vi "Controlled voltage ramp checking current.vi"(8 "V Ch 1":refnum<vi>, 9 "V Ch 0":refnum<vi>, 10 "Barcodes in":string[](array[string]), 11 "VISA Refnum in":refnum<visa-resource-name>) -> (0 "Ch 4 High":dbl[](array[numeric]), 1 "Ch 3 High":dbl[](array[numeric]), 2 "Ch 2 High":dbl[](array[numeric]), 3 "Ch 1 High":dbl[](array[numeric]), 4 "error out":errorcluster, 5 "BoardHandle out 3":T1, 6 "Current High":bool, 7 "Power Trip":bool)   [LabVIEW 2020]
uses:
  <instrlib>/CAEN PSM/CAEN PSM.lvlib
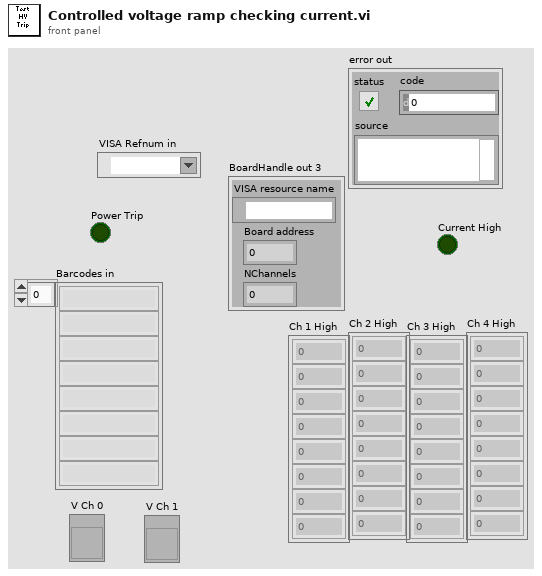
[diagram p1: front panel]
types:
  T1 = cluster{"VISA resource name":refnum<visa-resource-name>, "Board address":u8, "NChannels":u8}
  T2 = typedef "CAEN PSM.lvlib/BoardHandle.ctl" = cluster{"VISA resource name":refnum<visa-resource-name>, "Board address":i8, "NChannels":u8}
  T3 = cluster{"ON":bool, "RUP":bool, "RDW":bool, "OVC":bool, "OVV":bool, "UNV":bool, "MAXV":bool, "TRIP":bool, "OVP":bool, "OVT":bool, "DIS":bool, "KILL":bool, "ILK":bool, "NOCAL":bool}[]
  T4 = cluster{"ON":bool, "RUP":bool, "RDW":bool, "OVC":bool, "OVV":bool, "UNV":bool, "MAXV":bool, "TRIP":bool, "OVP":bool, "OVT":bool, "DIS":bool, "KILL":bool, "ILK":bool, "NOCAL":bool}
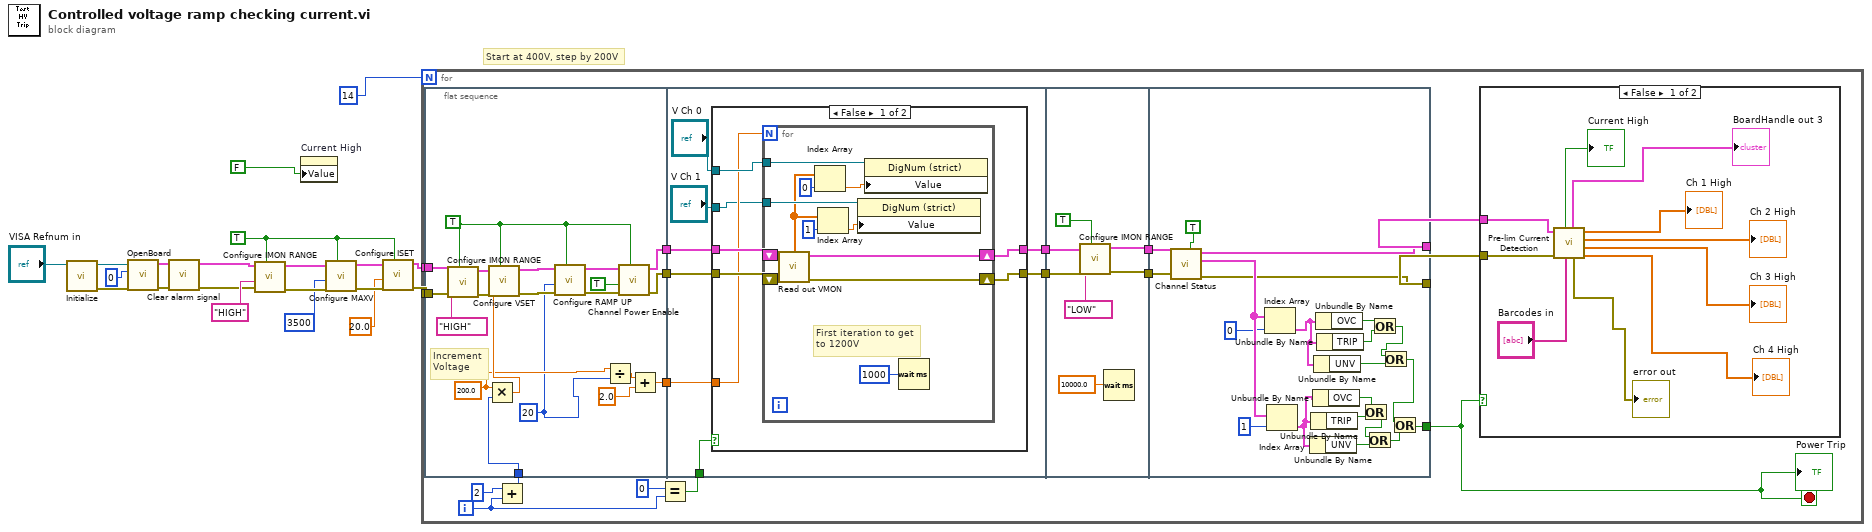
[diagram p0: block diagram]
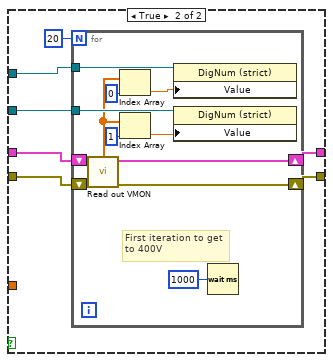
[diagram p3: hidden frame]
diagram:
  w6 = TRUE ("All Channels (F)")
  # "Start at 400V, step by 200V"
  n1 = call <instrlib>:"Initialize.vi"("VISA resource name"="VISA Refnum in") -> ("error out"=w17:errorcluster, "VISA resource name out"=w18:refnum<visa-resource-name>)  [unwired: 9 in]
  n2 = call <instrlib>:"OpenBoard.vi"("error in (no error)"=w17, "Board Address"=u8 0, "VISA resource name"=w18) -> ("error out"=w16:errorcluster, "BoardHandle"=w19:T2)  [unwired: 7 in]
  n3 = call <instrlib>:"Clear alarm signal.vi"("error in (no error)"=w16, "BoardHandle"=w19) -> ("error out"=w11:errorcluster, "BoardHandle out"=w12:T2)  [unwired: 8 in]
  n4 = call <instrlib>:"Configure IMON RANGE.vi"("All Channels (F)"=w6, "error in (no error)"=w11, "IMon range (LOW)"="HIGH", "BoardHandle"=w12) -> ("error out"=w9:errorcluster, "BoardHandle out"=w10:T2)  [unwired: 6 in]
  n5 = property on="Current High" class="Bool (strict)"("Value"=FALSE ("Current High")) -> ()  [unwired: 2 in, 2 out]
  n6 = call <instrlib>:"Configure MAXV.vi"("All Channels (F)"=w6, "error in (no error)"=w9, "Voltage Max (0.0 V)"=u16 3500, "BoardHandle"=w10) -> ("error out"=w7:errorcluster, "BoardHandle out"=w8:T2)  [unwired: 6 in]
  n7 = call <instrlib>:"Configure ISET.vi"("All Channels (F)"=w6, "error in (no error)"=w7, "Current Limit (0.00 uA)"=sgl 20.0, "BoardHandle"=w8) -> ("error out"=w4:errorcluster, "BoardHandle out"=w5:T2)  [unwired: 6 in]
  n8 = for {
    N: 14 -> [_]
    tunnel: w4 -> [w35]
    tunnel: w5 -> [w34]
    i -> [w27]
    stop <- w22 stop-if-true
    n9 = flat-sequence {
      tunnel: [w63] -> w37
      tunnel: [w62] -> w36
      tunnel: w30 -> [w59]
      tunnel: w35 -> [w57]
      tunnel: w34 -> [w58]
      tunnel: [w48] -> w21
      tunnel: w37 -> [w74]
      tunnel: w36 -> [w73]
      tunnel: [w72] -> w33
      tunnel: [w71] -> w32
      tunnel: w25 -> [w75]
      tunnel: w21 -> [w69]
      tunnel: w33 -> [w120]
      tunnel: [w117] -> w29
      tunnel: w32 -> [w119]
      tunnel: [w116] -> w28
      tunnel: w29 -> [w132]
      tunnel: w28 -> [w131]
      tunnel: [w133] -> w22
      tunnel: [w130] -> w24
      tunnel: [w129] -> w23
      frame #0 {
        w51 = u16 20 ("Voltage ramp up (0 V/s)")
        w52 = 200.0 ("x")
        w53 = TRUE ("All Channels (F)")
        # "Increment\nVoltage"
        n10 = call <instrlib>:"Configure IMON RANGE.vi"("All Channels (F)"=w53, "error in (no error)"=w57, "IMon range (LOW)"="HIGH", "BoardHandle"=w58) -> ("error out"=w56:errorcluster, "BoardHandle out"=w55:T2)  [unwired: 6 in]
        n11 = Multiply(x=w52, y=w59) -> (x*y=w60:dbl)
        n12 = call <instrlib>:"Configure VSET.vi"("All Channels (F)"=w53, "error in (no error)"=w56, "Voltage Level (0.0 V)"=w60, "BoardHandle"=w55) -> ("error out"=w66:errorcluster, "BoardHandle out"=w65:T2)  [unwired: 6 in]
        n13 = call <instrlib>:"Configure RAMP UP.vi"("All Channels (F)"=w53, "error in (no error)"=w66, "Voltage ramp up (0 V/s)"=w51, "BoardHandle"=w65) -> ("error out"=w67:errorcluster, "BoardHandle out"=w64:T2)  [unwired: 6 in]
        n14 = Divide(x=w52, y=w51) -> (x/y=w49:dbl)
        n15 = call <instrlib>:"Channel Power Enable.vi"("All Channels (F)"=w53, "error in (no error)"=w67, "Enable (OFF)"=TRUE ("Boolean"), "BoardHandle"=w64) -> ("error out"=w62:errorcluster, "BoardHandle out"=w63:T2)  [unwired: 6 in]
        n16 = Add(x=w49, y=2.0) -> (x+y=w48:dbl)
      }
      frame #1 {
        n17 = case shown="False" w75 {
          tunnel: w74 -> [w80 w101]
          tunnel: w73 -> [w79 w100]
          tunnel: [w82 w99] -> w72
          tunnel: [w81 w98] -> w71
          tunnel: "V Ch 0" -> [w78 w96]
          tunnel: w69 -> [w77 _]
          tunnel: "V Ch 1" -> [w76 w95]
          frame False {
            n18 = for {
              N: w77 -> [_]
              shift-right: [w91] -> w82
              shift-left: w80 -> [w93]
              shift-right: [w90] -> w81
              shift-left: w79 -> [w92]
              tunnel: w78 -> [w87]
              tunnel: w76 -> [w85]
              # "First iteration to get\nto 1200V"
              n19 = call <instrlib>:"Read out VMON.vi"("error in (no error)"=w92, "BoardHandle"=w93) -> ("error out"=w90:errorcluster, "VMon values (V)"=w83:dbl[], "BoardHandle out"=w91:T2)  [unwired: 7 in]
              n20 = Index Array(array=w83, index=0) -> (element=w88:dbl)
              n21 = Index Array(array=w83, index=1) -> (element=w84:dbl)
              n22 = property class="DigNum (strict)"(reference=w85, "Value"=w84) -> ()  [unwired: 1 in, 2 out]
              n23 = property class="DigNum (strict)"(reference=w87, "Value"=w88) -> ()  [unwired: 1 in, 2 out]
              n24 = Wait (ms)(milliseconds to wait=u32 1000) -> ()  [unwired: 1 out]
            }
          }
          frame True {
            n25 = for {
              N: 20 -> [_]
              shift-right: [w110] -> w99
              shift-left: w101 -> [w112]
              shift-right: [w109] -> w98
              shift-left: w100 -> [w111]
              tunnel: w96 -> [w106]
              tunnel: w95 -> [w104]
              # "First iteration to get\nto 400V"
              n26 = call <instrlib>:"Read out VMON.vi"("error in (no error)"=w111, "BoardHandle"=w112) -> ("error out"=w109:errorcluster, "VMon values (V)"=w102:dbl[], "BoardHandle out"=w110:T2)  [unwired: 7 in]
              n27 = Index Array(array=w102, index=0) -> (element=w107:dbl)
              n28 = Index Array(array=w102, index=1) -> (element=w103:dbl)
              n29 = property class="DigNum (strict)"(reference=w106, "Value"=w107) -> ()  [unwired: 1 in, 2 out]
              n30 = property class="DigNum (strict)"(reference=w104, "Value"=w103) -> ()  [unwired: 1 in, 2 out]
              n31 = Wait (ms)(milliseconds to wait=u32 1000) -> ()  [unwired: 1 out]
            }
          }
        }
      }
      frame #2 {
        n32 = call <instrlib>:"Configure IMON RANGE.vi"("All Channels (F)"=TRUE, "error in (no error)"=w119, "IMon range (LOW)"="LOW", "BoardHandle"=w120) -> ("error out"=w116:errorcluster, "BoardHandle out"=w117:T2)  [unwired: 6 in]
        n33 = Wait (ms)(milliseconds to wait=10000.0 ("x")) -> ()  [unwired: 1 out]
      }
      frame #3 {
        n34 = call <instrlib>:"Channel Status.vi"("All Channels (T)"=TRUE, "error in (no error)"=w131, "BoardHandle"=w132) -> ("error out"=w129:errorcluster, "Channel Status Array"=w141:T3, "BoardHandle out"=w130:T2)  [unwired: 5 in, 1 out]
        n35 = Index Array(array=w141, index=0) -> (element=w128:T4)
        n36 = Index Array(array=w141, index=1) -> (element=w124:T4)
        n37 = Unbundle By Name(w124) -> ("UNV"=w123:bool)
        n38 = Unbundle By Name(w124) -> ("TRIP"=w139:bool)
        n39 = Unbundle By Name(w124) -> ("OVC"=w140:bool)
        n40 = Unbundle By Name(w128) -> ("UNV"=w126:bool)
        n41 = Unbundle By Name(w128) -> ("OVC"=w138:bool)
        n42 = Unbundle By Name(w128) -> ("TRIP"=w137:bool)
        n43 = Or(x=w140, y=w139) -> (x .or. y?=w121:bool)
        n44 = Or(x=w121, y=w123) -> (x .or. y?=w122:bool)
        n45 = Or(x=w138, y=w137) -> (x .or. y?=w127:bool)
        n46 = Or(x=w127, y=w126) -> (x .or. y?=w125:bool)
        n47 = Or(x=w125, y=w122) -> (x .or. y?=w133:bool)
      }
    }
    n48 = Add(x=2, y=w27) -> (x+y=w30:i32)
    n49 = Equal?(x=0, y=w27) -> (x = y?=w25:bool)
    n50 = case shown="False" w22 {
      tunnel: w24 -> [w39 _]
      tunnel: w23 -> [w38 _]
      frame False {
        n51 = call "Pre-lim Current Detection.vi"("Barcodes in"="Barcodes in", "error in (no error)"=w38, "BoardHandle in 5"=w39) -> ("Ch 4 High"=→"Ch 4 High":dbl[], "Ch 3 High"=→"Ch 3 High":dbl[], "Ch 2 High"=→"Ch 2 High":dbl[], "Ch 1 High"=→"Ch 1 High":dbl[], "error out"=→"error out":errorcluster, "BoardHandle out 3"=→"BoardHandle out 3":T1, "Current High"=→"Current High":bool)  [unwired: 2 in]
      }
      frame True {
      }
    }
    "Power Trip" <- w22
  }
